vi "Botones_intensidad_txt.vi"(2 "Seleción método":bool, 8 "String":string, 9 "Array":dbl[](array[numeric]), 10 "Directorio scripts matlab 2":path=path "C:/Users/franjas/Documents/rutinas-calibracion-slm", 11 "I1":bool) -> (3 "?":bool)   [LabVIEW 2013]
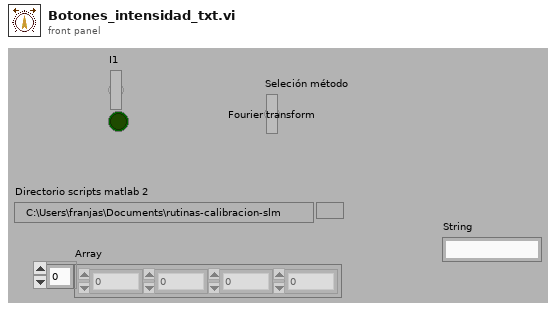
[diagram p1: front panel]
types:
  T1 = enum16{"Escritura", "Med fas", "Conf fase", "Med ampl", "Conf final", "finalizar"}
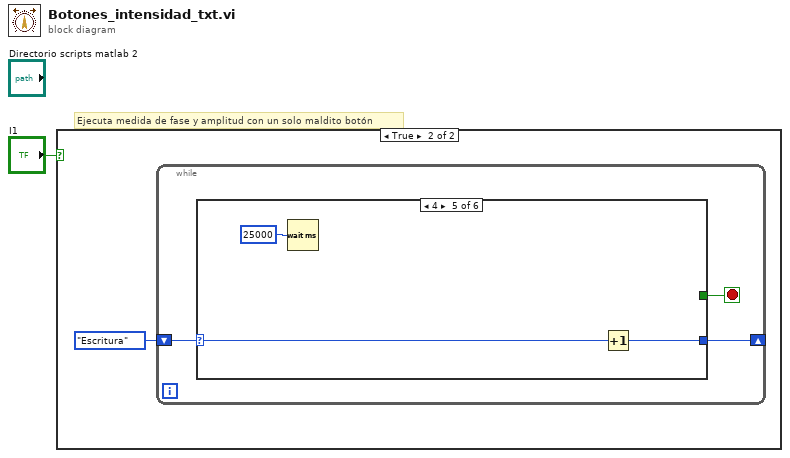
[diagram p0: block diagram]
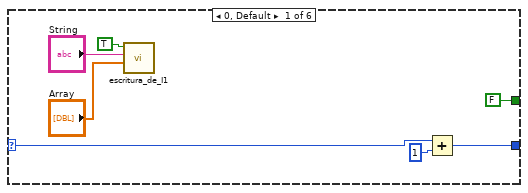
[diagram p3: hidden frame]
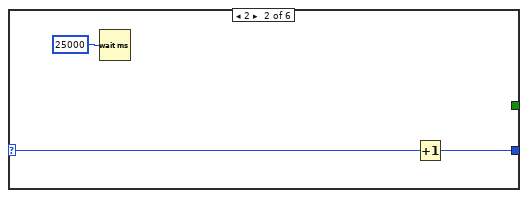
[diagram p4: hidden frame]
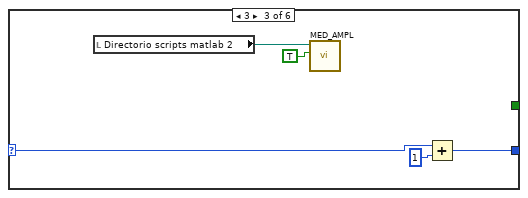
[diagram p5: hidden frame]
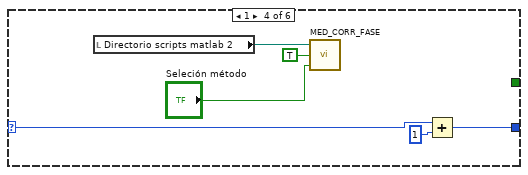
[diagram p6: hidden frame]
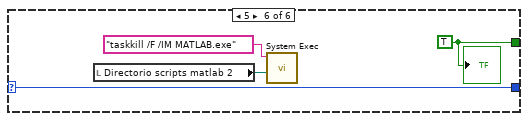
[diagram p7: hidden frame]
diagram:
  # "Ejecuta medida de fase y amplitud con un solo maldito botón"
  n1 = case shown="True" "I1" {
    frame False {
    }
    frame True {
      n2 = while {
        shift-right: [w4] -> _
        shift-left: T1."Escritura" -> [w5]
        stop <- w3 stop-if-true
        n3 = case shown="4" w5 {
          selector: w5 -> [w11 w13 w19 w25 w27 w32]
          tunnel: [w12 w14 w18 w24 w28 w32] -> w4
          tunnel: [FALSE ("I1\n<0,0|0,0>") _ _ _ _ w33] -> w3
          frame 0, Default {
            n4 = call "escritura_de_I1.vi"("I1\n<0,0|0,0>"=TRUE ("I1\n<0,0|0,0>"), "String"="String", "Array"="Array") -> ()  [unwired: 8 in]
            n5 = Add(x=w11, y=1) -> (x+y=w12:i32)
          }
          frame 2 {
            n6 = Wait (ms)(milliseconds to wait=u32 25000) -> ()  [unwired: 1 out]
            n7 = Increment(x=w13) -> (x+1=w14:i32)
          }
          frame 3 {
            n8 = local read "Directorio scripts matlab 2"() -> (w17:path)
            n9 = call "MED_AMPL.vi"("Boolean"=TRUE, "Directorio scripts matlab"=w17) -> ()  [unwired: 10 in]
            n10 = Add(x=w19, y=1) -> (x+y=w18:i32)
          }
          frame 1 {
            n11 = local read "Directorio scripts matlab 2"() -> (w23:path)
            n12 = call "MED_CORR_FASE.vi"("Seleción método"="Seleción método", "Ejecucion"=TRUE, "Directorio scripts matlab"=w23) -> ()
            n13 = Add(x=w25, y=1) -> (x+y=w24:i32)
          }
          frame 4 {
            n14 = Wait (ms)(milliseconds to wait=u32 25000) -> ()  [unwired: 1 out]
            n15 = Increment(x=w27) -> (x+1=w28:i32)
          }
          frame 5 {
            w33 = TRUE
            n16 = local read "Directorio scripts matlab 2"() -> (w30:path)
            n17 = call <vilib>:"System Exec.vi"("working directory"=w30, "command line"="taskkill /F /IM MATLAB.exe") -> ()  [unwired: 6 in, 4 out]
            "?" <- w33
          }
        }
      }
    }
  }
